vi "Crossover.vi"(9 "Boolean 2":bool, 10 "Numeric in":dbl, 11 "Boolean":bool) -> (3 "Numeric out":dbl)   [LabVIEW 2017]
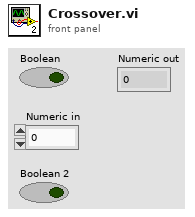
[diagram p1: front panel]
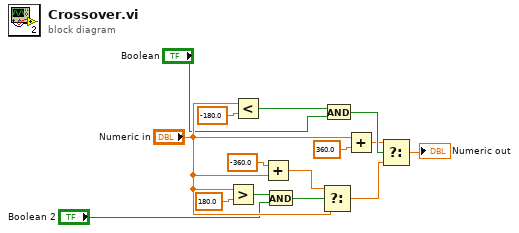
[diagram p0: block diagram]
diagram:
  n1 = Greater?(x="Numeric in", y=180.0) -> (0:w6:bool)
  n2 = Less?(x="Numeric in", y=-180.0) -> (x < y?=w12:bool)
  n3 = Add(x=-360.0, y="Numeric in") -> (x+y=w3:dbl)
  n4 = And(x=w6, y="Boolean 2") -> (x .and. y?=w5:bool)
  n5 = Select(t=w3, s=w5, f="Numeric in") -> (s? t:f=w2:dbl)
  n6 = And(x=w12, y="Boolean") -> (x .and. y?=w11:bool)
  n7 = Add(x="Numeric in", y=360.0) -> (x+y=w9:dbl)
  n8 = Select(t=w9, s=w11, f=w2) -> (s? t:f=→"Numeric out":dbl)
